vi "Simulator.vi"(6 "Proportions":dbl[](array[numeric]), 8 "Delays (s)":dbl[](array[numeric]) format="%#_9g", 9 "Active Channels":T1={"A="=FALSE, "B="=FALSE, "C="=TRUE, "D="=TRUE}, 11 "Calibration":dbl[][](array[numeric])=[[0.000303, 0.000306, 0.000498714, 0.000498713, 0.05], [0.000303, 0.000306, 0.000499714, 0.000499713, 0.1], [0.000303, 0.000306, 0.000500314, 0.000500413, 0.2], [0.000303, 0.000306, 0.000501314, 0.000501413, 0.5], [0.000303, 0.000306, 0.000501914, 0.000501813, 1.0], [0.000303, 0.000306, 0.000502414, 0.000502213, 2.0], [0.000303, 0.000306, 0.000502514, 0.000502513, 3.0], [0.000303, 0.000306, 0.000502714, 0.000502613, 4.0], [0.000303, 0.000306, 0.000502914, 0.000502813, 5.0], [0.000303, 0.000306, 0.000503014, 0.000503013, 6.1], [0.000303, 0.000306, 0.000503114, 0.000503113, 7.0], [0.000303, 0.000306, 0.000503214, 0.000503213, 8.0], [0.000303, 0.000306, 0.000503314, 0.000503313, 9.0], [0.000303, 0.000306, 0.000503314, 0.000503413, 9.7]]) -> (0 "Output Energy (J)":dbl, 3 "Output Power (W)":dbl)   [LabVIEW 2009]
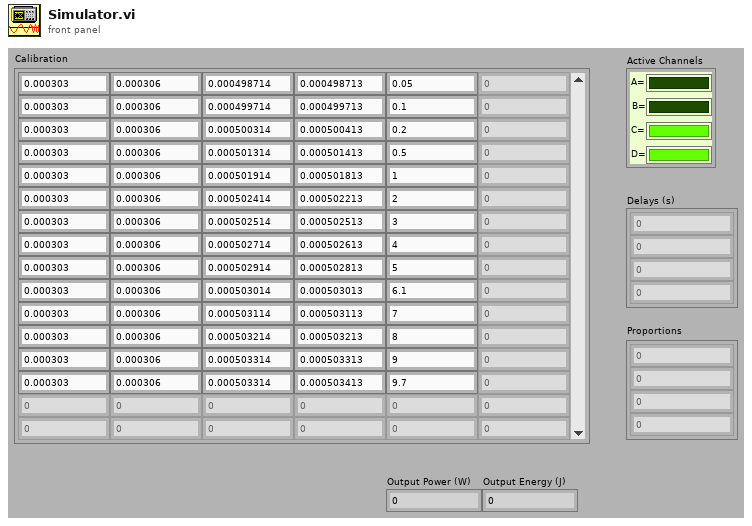
[diagram p1: front panel]
types:
  T1 = cluster{"A=":bool, "B=":bool, "C=":bool, "D=":bool}
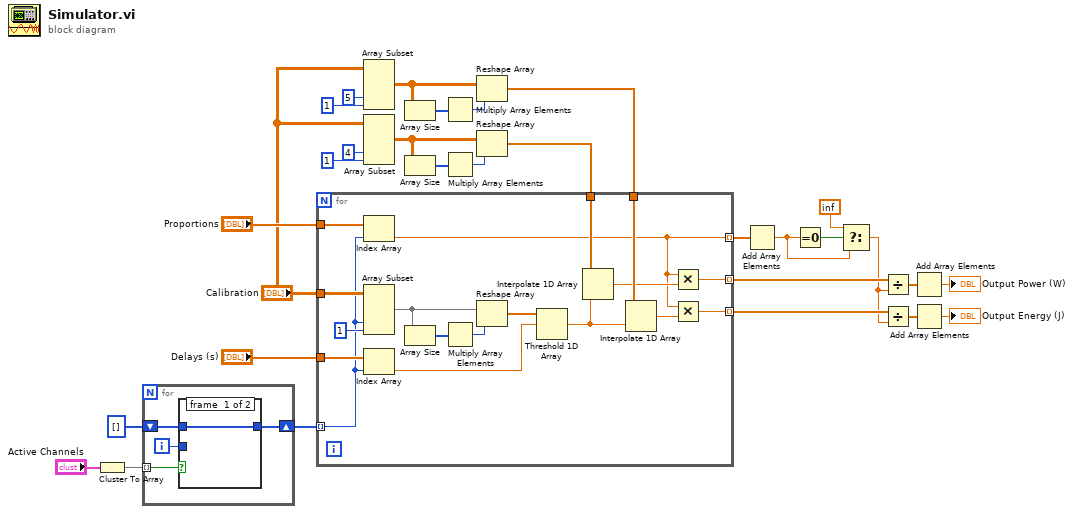
[diagram p0: block diagram]
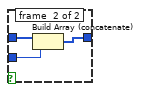
[diagram p2: hidden frame]
diagram:
  n1 = Cluster To Array(cluster="Active Channels") -> (array=w3:bool[])
  n2 = for {
    tunnel: w3 -> [w34] mode=indexing
    shift-right: [w31] -> w1
    shift-left: i32[] [] -> [w33]
    i -> [w32]
    n3 = case shown="True" w34 {
      tunnel: w33 -> [w35 w38]
      tunnel: w32 -> [_ w37]
      tunnel: [w35 w36] -> w31
      frame #0 {
      }
      frame #1 {
        n4 = Build Array (concatenate)(w38, w37) -> (w36:i32[])
      }
    }
  }
  n5 = Array Subset(array="Calibration", index (col)=5 ("index"), length (col)=1 ("length")) -> (w27:dbl[][])  [unwired: 2 in]
  n6 = Array Subset(array="Calibration", index (col)=4 ("index"), length (col)=1 ("length")) -> (w20:dbl[][])  [unwired: 2 in]
  n7 = Array Size(array=w27) -> (size(s)=w26:i32[])
  n8 = Array Size(array=w20) -> (size(s)=w21:i32[])
  n9 = Multiply Array Elements(1:w26) -> (0:w28:i32)
  n10 = Multiply Array Elements(1:w21) -> (0:w19:i32)
  n11 = Reshape Array(w27, w28) -> (w16:dbl[])
  n12 = Reshape Array(w20, w19) -> (w17:dbl[])
  n13 = for {
    tunnel: w1 -> [w49] mode=indexing
    tunnel: "Delays (s)" -> [w56]
    tunnel: "Calibration" -> [w55]
    tunnel: "Proportions" -> [w50]
    tunnel: w17 -> [w45]
    tunnel: w16 -> [w44]
    tunnel: [w41] -> w14 mode=indexing
    tunnel: [w40] -> w13 mode=indexing
    tunnel: [w39] -> w15 mode=indexing
    n14 = Index Array(array=w50, index=w49) -> (element=w39:dbl)
    n15 = Array Subset(array=w55, index (col)=w49, length (col)=1 ("length")) -> (w52:dbl[][])  [unwired: 2 in]
    n16 = Index Array(array=w56, index=w49) -> (element=w47:dbl)
    n17 = Array Size(array=w52) -> (size(s)=w53:i32[])
    n18 = Multiply Array Elements(1:w53) -> (0:w51:i32)
    n19 = Reshape Array(w52, w51) -> (w48:dbl[])
    n20 = Threshold 1D Array(2:w47, 3:w48) -> (0:w46:dbl)  [unwired: 1 in]
    n21 = Interpolate 1D Array(1:w46, 2:w45) -> (0:w43:dbl)
    n22 = Interpolate 1D Array(1:w46, 2:w44) -> (0:w42:dbl)
    n23 = Multiply(x=w39, y=w43) -> (x*y=w41:dbl)
    n24 = Multiply(x=w39, y=w42) -> (x*y=w40:dbl)
  }
  n25 = Add Array Elements(numeric array=w15) -> (sum=w7:dbl)
  n26 = Equal To 0?(x=w7) -> (x = 0?=w8:bool)
  n27 = Select(t=inf, s=w8, f=w7) -> (s? t:f=w5:dbl)
  n28 = Divide(x=w14, y=w5) -> (x/y=w12:dbl[])
  n29 = Divide(x=w13, y=w5) -> (x/y=w11:dbl[])
  n30 = Add Array Elements(numeric array=w12) -> (sum=→"Output Power (W)":dbl)
  n31 = Add Array Elements(numeric array=w11) -> (sum=→"Output Energy (J)":dbl)
